vi "FuzzyEx User-defined Membership Functions.vi"() -> ()   [LabVIEW 2023]
doc: "This VI demonstrates how to create your own user-defined membership function and use the API to evaluate a system by using the new membership function."
uses:
  <vilib>/addons/Fuzzy Logic/TypeDefs/FL Modifier.ctl
  <vilib>/addons/Fuzzy Logic/TypeDefs/FL Antecedent Connective.ctl
  <vilib>/addons/Fuzzy Logic/TypeDefs/FL Consequent Implication.ctl
  <vilib>/addons/Fuzzy Logic/Membership/FL Create Membership Function (User-Defined).vi
  <vilib>/addons/Fuzzy Logic/FL Fuzzy Controller (SISO).vi
  <vilib>/addons/Fuzzy Logic/NI_Fuzzy_Logic_API.lvlib
panel:
  in  "Overview":string="Overview: This VI demonstrates how to create your own user-defined membership function and use the API to evaluate a system by using the new membership function.\nInstructions:\n1. Run the VI.\n2. Change shape by moving the Basic Membership Shape cursors or directly changing values in the cursor table. Keep in mind the X and Y arrays must contain elements in ascending order for convenient interpolation results. \n3. Move the slider below the Membership Function graph to evaluate the membership grade.\n4. Change the left base, left top, right top and right base values to modify the range of the function.\n5. Click Stop to stop the VI."
  out "Error":bool
  in  "Basic Membership Shape":cluster{cluster{"Xi":dbl, "Yi":dbl}[]}[](graph)=[{[{"Xi"=-8.0, "Yi"=0.0}, {"Xi"=-7.919597989949748, "Yi"=0.04719031897891056}, {"Xi"=-7.839195979899498, "Yi"=0.0936509941538288}, {"Xi"=-7.758793969849246, "Yi"=0.13877501021805186}, {"Xi"=-7.678391959798995, "Yi"=0.18195535186487483}, {"Xi"=-7.597989949748744, "Yi"=0.22258500378759477}, {"Xi"=-7.517587939698492, "Yi"=0.26039081912974815}, {"Xi"=-7.437185929648241, "Yi"=0.29776297115463546}, {"Xi"=-7.35678391959799, "Yi"=0.3351151121007157}, {"Xi"=-7.276381909547739, "Yi"=0.37222372887356214}, {"Xi"=-7.1959798994974875, "Yi"=0.4088653083787497}, {"Xi"=-7.115577889447236, "Yi"=0.44481633752185185}, {"Xi"=-7.035175879396985, "Yi"=0.4798533032084424}, {"Xi"=-6.954773869346734, "Yi"=0.513752692344096}, {"Xi"=-6.874371859296482, "Yi"=0.5462909918343865}, {"Xi"=-6.793969849246231, "Yi"=0.5772446885848874}, {"Xi"=-6.71356783919598, "Yi"=0.6063902695011735}, {"Xi"=-6.633165829145729, "Yi"=0.6335042214888181}, {"Xi"=-6.552763819095477, "Yi"=0.6583630314533961}, {"Xi"=-6.472361809045226, "Yi"=0.6807431863004809}, {"Xi"=-6.391959798994975, "Yi"=0.7004211729356467}, {"Xi"=-6.311557788944723, "Yi"=0.7172252080175027}, {"Xi"=-6.231155778894473, "Yi"=0.7329213118498933}, {"Xi"=-6.150753768844221, "Yi"=0.7484474478322185}, {"Xi"=-6.0703517587939695, "Yi"=0.7637753085739313}, {"Xi"=-5.989949748743719, "Yi"=0.7788765866844846}, {"Xi"=-5.909547738693467, "Yi"=0.7937229747733321}, {"Xi"=-5.8291457286432165, "Yi"=0.8082861654499267}, {"Xi"=-5.748743718592965, "Yi"=0.8225378513237219}, {"Xi"=-5.668341708542713, "Yi"=0.8364497250041708}, {"Xi"=-5.5879396984924625, "Yi"=0.8499934791007266}, {"Xi"=-5.507537688442211, "Yi"=0.8631408062228427}, {"Xi"=-5.42713567839196, "Yi"=0.875863398979972}, {"Xi"=-5.346733668341709, "Yi"=0.8881329499815682}, {"Xi"=-5.266331658291457, "Yi"=0.8999211518370842}, {"Xi"=-5.185929648241206, "Yi"=0.9111996971559733}, {"Xi"=-5.105527638190955, "Yi"=0.9219402785476887}, {"Xi"=-5.025125628140704, "Yi"=0.9321145886216837}, {"Xi"=-4.944723618090452, "Yi"=0.9416943199874116}, {"Xi"=-4.864321608040201, "Yi"=0.9506511652543255}, {"Xi"=-4.78391959798995, "Yi"=0.9589568170318786}, {"Xi"=-4.703517587939698, "Yi"=0.9665829679295244}, {"Xi"=-4.623115577889447, "Yi"=0.9735013105567158}, {"Xi"=-4.542713567839196, "Yi"=0.9796835375229063}, {"Xi"=-4.4623115577889445, "Yi"=0.985101341437549}, {"Xi"=-4.381909547738694, "Yi"=0.989726414910097}, {"Xi"=-4.301507537688442, "Yi"=0.993530450550004}, {"Xi"=-4.221105527638191, "Yi"=0.9964851409667227}, {"Xi"=-4.14070351758794, "Yi"=0.9985621787697065}, {"Xi"=-4.060301507537688, "Yi"=0.9997332565684088}, {"Xi"=-3.979899497487437, "Yi"=1.0}, {"Xi"=-3.899497487437186, "Yi"=1.0}, {"Xi"=-3.819095477386935, "Yi"=1.0}, {"Xi"=-3.7386934673366836, "Yi"=1.0}, {"Xi"=-3.658291457286432, "Yi"=1.0}, {"Xi"=-3.577889447236181, "Yi"=1.0}, {"Xi"=-3.4974874371859297, "Yi"=1.0}, {"Xi"=-3.4170854271356785, "Yi"=1.0}, {"Xi"=-3.336683417085427, "Yi"=1.0}, {"Xi"=-3.2562814070351758, "Yi"=1.0}, {"Xi"=-3.1758793969849246, "Yi"=1.0}, {"Xi"=-3.0954773869346734, "Yi"=1.0}, {"Xi"=-3.0150753768844223, "Yi"=1.0}, {"Xi"=-2.9346733668341707, "Yi"=1.0}, {"Xi"=-2.8542713567839195, "Yi"=1.0}, {"Xi"=-2.7738693467336684, "Yi"=1.0}, {"Xi"=-2.693467336683417, "Yi"=1.0}, {"Xi"=-2.613065326633166, "Yi"=1.0}, {"Xi"=-2.5326633165829144, "Yi"=1.0}, {"Xi"=-2.4522613065326633, "Yi"=1.0}, {"Xi"=-2.371859296482412, "Yi"=1.0}, {"Xi"=-2.291457286432161, "Yi"=1.0}, {"Xi"=-2.2110552763819094, "Yi"=1.0}, {"Xi"=-2.130653266331658, "Yi"=1.0}, {"Xi"=-2.050251256281407, "Yi"=1.0}, {"Xi"=-1.9698492462311559, "Yi"=1.0}, {"Xi"=-1.8894472361809045, "Yi"=1.0}, {"Xi"=-1.8090452261306533, "Yi"=1.0}, {"Xi"=-1.728643216080402, "Yi"=1.0}, {"Xi"=-1.6482412060301508, "Yi"=1.0}, {"Xi"=-1.5678391959798994, "Yi"=1.0}, {"Xi"=-1.4874371859296482, "Yi"=1.0}, {"Xi"=-1.407035175879397, "Yi"=1.0}, {"Xi"=-1.3266331658291457, "Yi"=1.0}, {"Xi"=-1.2462311557788945, "Yi"=1.0}, {"Xi"=-1.1658291457286432, "Yi"=1.0}, {"Xi"=-1.085427135678392, "Yi"=1.0}, {"Xi"=-1.0050251256281406, "Yi"=1.0}, {"Xi"=-0.9246231155778895, "Yi"=1.0}, {"Xi"=-0.8442211055276382, "Yi"=1.0}, {"Xi"=-0.7638190954773869, "Yi"=1.0}, {"Xi"=-0.6834170854271356, "Yi"=1.0}, {"Xi"=-0.6030150753768844, "Yi"=1.0}, {"Xi"=-0.5226130653266332, "Yi"=1.0}, {"Xi"=-0.44221105527638194, "Yi"=1.0}, {"Xi"=-0.36180904522613067, "Yi"=1.0}, {"Xi"=-0.2814070351758794, "Yi"=1.0}, {"Xi"=-0.20100502512562815, "Yi"=1.0}, {"Xi"=-0.12060301507537688, "Yi"=1.0}, {"Xi"=-0.04020100502512563, "Yi"=1.0}, {"Xi"=0.04020100502512563, "Yi"=1.0}, {"Xi"=0.12060301507537688, "Yi"=1.0}, {"Xi"=0.20100502512562815, "Yi"=1.0}, {"Xi"=0.2814070351758794, "Yi"=1.0}, {"Xi"=0.36180904522613067, "Yi"=1.0}, {"Xi"=0.44221105527638194, "Yi"=1.0}, {"Xi"=0.5226130653266332, "Yi"=1.0}, {"Xi"=0.6030150753768844, "Yi"=1.0}, {"Xi"=0.6834170854271356, "Yi"=1.0}, {"Xi"=0.7638190954773869, "Yi"=1.0}, {"Xi"=0.8442211055276382, "Yi"=1.0}, {"Xi"=0.9246231155778895, "Yi"=1.0}, {"Xi"=1.0050251256281406, "Yi"=0.999999390841234}, {"Xi"=1.085427135678392, "Yi"=0.9998249469013698}, {"Xi"=1.1658291457286432, "Yi"=0.9993441155957051}, {"Xi"=1.2462311557788945, "Yi"=0.9985621787697065}, {"Xi"=1.3266331658291457, "Yi"=0.9974844182688406}, {"Xi"=1.407035175879397, "Yi"=0.9961161159385735}, {"Xi"=1.4874371859296482, "Yi"=0.994462553624372}, {"Xi"=1.5678391959798994, "Yi"=0.9925290131717022}, {"Xi"=1.6482412060301508, "Yi"=0.9903207764260309}, {"Xi"=1.728643216080402, "Yi"=0.9878431252328242}, {"Xi"=1.8090452261306533, "Yi"=0.985101341437549}, {"Xi"=1.8894472361809045, "Yi"=0.9821007068856714}, {"Xi"=1.9698492462311559, "Yi"=0.9788465034226579}, {"Xi"=2.050251256281407, "Yi"=0.975344012893975}, {"Xi"=2.130653266331658, "Yi"=0.9715985171450893}, {"Xi"=2.2110552763819094, "Yi"=0.967615298021467}, {"Xi"=2.291457286432161, "Yi"=0.9633996373685746}, {"Xi"=2.371859296482412, "Yi"=0.9589568170318786}, {"Xi"=2.4522613065326633, "Yi"=0.9542921188568456}, {"Xi"=2.5326633165829144, "Yi"=0.9494108246889419}, {"Xi"=2.613065326633166, "Yi"=0.9443182163736339}, {"Xi"=2.693467336683417, "Yi"=0.9390195757563881}, {"Xi"=2.7738693467336684, "Yi"=0.9335201846826711}, {"Xi"=2.8542713567839195, "Yi"=0.927825324997949}, {"Xi"=2.9346733668341707, "Yi"=0.9219402785476887}, {"Xi"=3.0150753768844223, "Yi"=0.9158703271773563}, {"Xi"=3.0954773869346734, "Yi"=0.9096207527324184}, {"Xi"=3.1758793969849246, "Yi"=0.9031968370583415}, {"Xi"=3.2562814070351758, "Yi"=0.896603862000592}, {"Xi"=3.336683417085427, "Yi"=0.8898471094046363}, {"Xi"=3.4170854271356785, "Yi"=0.8829318611159407}, {"Xi"=3.4974874371859297, "Yi"=0.8758633989799721}, {"Xi"=3.577889447236181, "Yi"=0.8686470048421966}, {"Xi"=3.658291457286432, "Yi"=0.8612879605480808}, {"Xi"=3.7386934673366836, "Yi"=0.8537915479430909}, {"Xi"=3.819095477386935, "Yi"=0.8461630488726938}, {"Xi"=3.899497487437186, "Yi"=0.8384077451823555}, {"Xi"=3.979899497487437, "Yi"=0.8305309187175428}, {"Xi"=4.060301507537688, "Yi"=0.8225378513237219}, {"Xi"=4.14070351758794, "Yi"=0.8144338248463594}, {"Xi"=4.221105527638191, "Yi"=0.8062241211309217}, {"Xi"=4.301507537688442, "Yi"=0.7979140220228752}, {"Xi"=4.381909547738694, "Yi"=0.7895088093676864}, {"Xi"=4.4623115577889445, "Yi"=0.781013765010822}, {"Xi"=4.542713567839196, "Yi"=0.772434170797748}, {"Xi"=4.623115577889447, "Yi"=0.7637753085739312}, {"Xi"=4.703517587939698, "Yi"=0.7550424601848378}, {"Xi"=4.78391959798995, "Yi"=0.7462409074759343}, {"Xi"=4.864321608040201, "Yi"=0.7373759322926875}, {"Xi"=4.944723618090452, "Yi"=0.7284528164805634}, {"Xi"=5.025125628140704, "Yi"=0.7194768418850286}, {"Xi"=5.105527638190955, "Yi"=0.7103665016452464}, {"Xi"=5.185929648241206, "Yi"=0.7004211729356467}, {"Xi"=5.266331658291457, "Yi"=0.6895205197178526}, {"Xi"=5.346733668341709, "Yi"=0.6777062470590457}, {"Xi"=5.42713567839196, "Yi"=0.6650200600264075}, {"Xi"=5.507537688442211, "Yi"=0.6515036636871199}, {"Xi"=5.5879396984924625, "Yi"=0.6371987631083638}, {"Xi"=5.668341708542713, "Yi"=0.6221470633573212}, {"Xi"=5.748743718592965, "Yi"=0.6063902695011734}, {"Xi"=5.8291457286432165, "Yi"=0.5899700866071019}, {"Xi"=5.909547738693467, "Yi"=0.5729282197422885}, {"Xi"=5.989949748743719, "Yi"=0.5553063739739142}, {"Xi"=6.0703517587939695, "Yi"=0.5371462543691613}, {"Xi"=6.150753768844221, "Yi"=0.5184895659952105}, {"Xi"=6.231155778894473, "Yi"=0.49937801391924364}, {"Xi"=6.311557788944723, "Yi"=0.47985330320844255}, {"Xi"=6.391959798994975, "Yi"=0.45995713892998824}, {"Xi"=6.472361809045226, "Yi"=0.4397312261510627}, {"Xi"=6.552763819095477, "Yi"=0.419217269938847}, {"Xi"=6.633165829145729, "Yi"=0.3984569753605229}, {"Xi"=6.71356783919598, "Yi"=0.37749204748327214}, {"Xi"=6.793969849246231, "Yi"=0.3563641913742757}, {"Xi"=6.874371859296482, "Yi"=0.33511511210071576}, {"Xi"=6.954773869346734, "Yi"=0.31378651472977315}, {"Xi"=7.035175879396985, "Yi"=0.2924201043286298}, {"Xi"=7.115577889447236, "Yi"=0.2710575859644674}, {"Xi"=7.1959798994974875, "Yi"=0.24974066470446693}, {"Xi"=7.276381909547739, "Yi"=0.22814562572871505}, {"Xi"=7.35678391959799, "Yi"=0.2055235591010643}, {"Xi"=7.437185929648241, "Yi"=0.18195535186487494}, {"Xi"=7.517587939698492, "Yi"=0.1575542663514276}, {"Xi"=7.597989949748744, "Yi"=0.13243356489200173}, {"Xi"=7.678391959798995, "Yi"=0.1067065098178776}, {"Xi"=7.758793969849246, "Yi"=0.08048636346033558}, {"Xi"=7.839195979899498, "Yi"=0.053886388150655086}, {"Xi"=7.919597989949748, "Yi"=0.027019846220116755}, {"Xi"=8.0, "Yi"=0.0}]}]
  in  "Stop":bool
  out "Membership grade":dbl(slide)=0.6596021514020028 scale=0.0..1.0
  in  "input value":dbl(slide)=4.535315985130112 scale=-10.0..10.0
  out "Membership function":cluster{cluster{"Xi":dbl, "Yi":dbl}[]}[](graph)=[{[{"Xi"=-8.0, "Yi"=0.0}, {"Xi"=-7.919597989949748, "Yi"=0.04525637619716676}, {"Xi"=-7.839195979899498, "Yi"=0.089101739755963}, {"Xi"=-7.758793969849246, "Yi"=0.13147220499791226}, {"Xi"=-7.678391959798995, "Yi"=0.17230388624453624}, {"Xi"=-7.597989949748744, "Yi"=0.21153289781735835}, {"Xi"=-7.517587939698492, "Yi"=0.24909535403790078}, {"Xi"=-7.437185929648241, "Yi"=0.2849273692276857}, {"Xi"=-7.35678391959799, "Yi"=0.3189650577082365}, {"Xi"=-7.276381909547739, "Yi"=0.351144533801075}, {"Xi"=-7.1959798994974875, "Yi"=0.38140191182772454}, {"Xi"=-7.115577889447236, "Yi"=0.40967330610970726}, {"Xi"=-7.035175879396985, "Yi"=0.4358948309685456}, {"Xi"=-6.954773869346734, "Yi"=0.46000260072576254}, {"Xi"=-6.874371859296482, "Yi"=0.4819165744611297}, {"Xi"=-6.793969849246231, "Yi"=0.5016954632128382}, {"Xi"=-6.71356783919598, "Yi"=0.5197150776642824}, {"Xi"=-6.633165829145729, "Yi"=0.5363726915150068}, {"Xi"=-6.552763819095477, "Yi"=0.5520655784645572}, {"Xi"=-6.472361809045226, "Yi"=0.5671910122124783}, {"Xi"=-6.391959798994975, "Yi"=0.5821462664583151}, {"Xi"=-6.311557788944723, "Yi"=0.5973286149016133}, {"Xi"=-6.231155778894473, "Yi"=0.6131353312419173}, {"Xi"=-6.150753768844221, "Yi"=0.629955017725542}, {"Xi"=-6.0703517587939695, "Yi"=0.6479014267980455}, {"Xi"=-5.989949748743719, "Yi"=0.6668179425698928}, {"Xi"=-5.909547738693467, "Yi"=0.686538545391848}, {"Xi"=-5.8291457286432165, "Yi"=0.7068972156146747}, {"Xi"=-5.748743718592965, "Yi"=0.7277279335891373}, {"Xi"=-5.668341708542713, "Yi"=0.7488646796659998}, {"Xi"=-5.5879396984924625, "Yi"=0.7701414341960257}, {"Xi"=-5.507537688442211, "Yi"=0.7913921775299795}, {"Xi"=-5.42713567839196, "Yi"=0.8124508900186247}, {"Xi"=-5.346733668341709, "Yi"=0.8331515520127257}, {"Xi"=-5.266331658291457, "Yi"=0.8533281438630463}, {"Xi"=-5.185929648241206, "Yi"=0.8728146459203504}, {"Xi"=-5.105527638190955, "Yi"=0.8914450385354021}, {"Xi"=-5.025125628140704, "Yi"=0.9090533020589653}, {"Xi"=-4.944723618090452, "Yi"=0.9254734168418042}, {"Xi"=-4.864321608040201, "Yi"=0.9405393632346825}, {"Xi"=-4.78391959798995, "Yi"=0.9540851215883641}, {"Xi"=-4.703517587939698, "Yi"=0.9659446722536132}, {"Xi"=-4.623115577889447, "Yi"=0.9759519955811939}, {"Xi"=-4.542713567839196, "Yi"=0.9839410719218699}, {"Xi"=-4.4623115577889445, "Yi"=0.9897458816264053}, {"Xi"=-4.381909547738694, "Yi"=0.9932004074607601}, {"Xi"=-4.301507537688442, "Yi"=0.9953659353767574}, {"Xi"=-4.221105527638191, "Yi"=0.9972948938536792}, {"Xi"=-4.14070351758794, "Yi"=0.9988182838797}, {"Xi"=-4.060301507537688, "Yi"=0.9997671064429944}, {"Xi"=-3.979899497487437, "Yi"=1.0}, {"Xi"=-3.899497487437186, "Yi"=1.0}, {"Xi"=-3.819095477386935, "Yi"=1.0}, {"Xi"=-3.7386934673366836, "Yi"=1.0}, {"Xi"=-3.658291457286432, "Yi"=1.0}, {"Xi"=-3.577889447236181, "Yi"=1.0}, {"Xi"=-3.4974874371859297, "Yi"=1.0}, {"Xi"=-3.4170854271356785, "Yi"=1.0}, {"Xi"=-3.336683417085427, "Yi"=1.0}, {"Xi"=-3.2562814070351758, "Yi"=1.0}, {"Xi"=-3.1758793969849246, "Yi"=1.0}, {"Xi"=-3.0954773869346734, "Yi"=1.0}, {"Xi"=-3.0150753768844223, "Yi"=1.0}, {"Xi"=-2.9346733668341707, "Yi"=1.0}, {"Xi"=-2.8542713567839195, "Yi"=1.0}, {"Xi"=-2.7738693467336684, "Yi"=1.0}, {"Xi"=-2.693467336683417, "Yi"=1.0}, {"Xi"=-2.613065326633166, "Yi"=1.0}, {"Xi"=-2.5326633165829144, "Yi"=1.0}, {"Xi"=-2.4522613065326633, "Yi"=1.0}, {"Xi"=-2.371859296482412, "Yi"=1.0}, {"Xi"=-2.291457286432161, "Yi"=1.0}, {"Xi"=-2.2110552763819094, "Yi"=1.0}, {"Xi"=-2.130653266331658, "Yi"=1.0}, {"Xi"=-2.050251256281407, "Yi"=1.0}, {"Xi"=-1.9698492462311559, "Yi"=1.0}, {"Xi"=-1.8894472361809045, "Yi"=1.0}, {"Xi"=-1.8090452261306533, "Yi"=1.0}, {"Xi"=-1.728643216080402, "Yi"=1.0}, {"Xi"=-1.6482412060301508, "Yi"=1.0}, {"Xi"=-1.5678391959798994, "Yi"=1.0}, {"Xi"=-1.4874371859296482, "Yi"=1.0}, {"Xi"=-1.407035175879397, "Yi"=1.0}, {"Xi"=-1.3266331658291457, "Yi"=1.0}, {"Xi"=-1.2462311557788945, "Yi"=1.0}, {"Xi"=-1.1658291457286432, "Yi"=1.0}, {"Xi"=-1.085427135678392, "Yi"=1.0}, {"Xi"=-1.0050251256281406, "Yi"=1.0}, {"Xi"=-0.9246231155778895, "Yi"=1.0}, {"Xi"=-0.8442211055276382, "Yi"=1.0}, {"Xi"=-0.7638190954773869, "Yi"=1.0}, {"Xi"=-0.6834170854271356, "Yi"=1.0}, {"Xi"=-0.6030150753768844, "Yi"=1.0}, {"Xi"=-0.5226130653266332, "Yi"=1.0}, {"Xi"=-0.44221105527638194, "Yi"=1.0}, {"Xi"=-0.36180904522613067, "Yi"=1.0}, {"Xi"=-0.2814070351758794, "Yi"=1.0}, {"Xi"=-0.20100502512562815, "Yi"=1.0}, {"Xi"=-0.12060301507537688, "Yi"=1.0}, {"Xi"=-0.04020100502512563, "Yi"=1.0}, {"Xi"=0.04020100502512563, "Yi"=1.0}, {"Xi"=0.12060301507537688, "Yi"=1.0}, {"Xi"=0.20100502512562815, "Yi"=1.0}, {"Xi"=0.2814070351758794, "Yi"=1.0}, {"Xi"=0.36180904522613067, "Yi"=1.0}, {"Xi"=0.44221105527638194, "Yi"=1.0}, {"Xi"=0.5226130653266332, "Yi"=1.0}, {"Xi"=0.6030150753768844, "Yi"=1.0}, {"Xi"=0.6834170854271356, "Yi"=1.0}, {"Xi"=0.7638190954773869, "Yi"=1.0}, {"Xi"=0.8442211055276382, "Yi"=1.0}, {"Xi"=0.9246231155778895, "Yi"=1.0}, {"Xi"=1.0050251256281406, "Yi"=0.9999994462347956}, {"Xi"=1.085427135678392, "Yi"=0.9998458948873343}, {"Xi"=1.1658291457286432, "Yi"=0.9994416629878643}, {"Xi"=1.2462311557788945, "Yi"=0.9988182838797}, {"Xi"=1.3266331658291457, "Yi"=0.9980072909061556}, {"Xi"=1.407035175879397, "Yi"=0.9970402174105455}, {"Xi"=1.4874371859296482, "Yi"=0.9959485967361842}, {"Xi"=1.5678391959798994, "Yi"=0.9947639622263859}, {"Xi"=1.6482412060301508, "Yi"=0.9935178472244648}, {"Xi"=1.728643216080402, "Yi"=0.9920183336567963}, {"Xi"=1.8090452261306533, "Yi"=0.9897458816264053}, {"Xi"=1.8894472361809045, "Yi"=0.9867059891762994}, {"Xi"=1.9698492462311559, "Yi"=0.9829296337337414}, {"Xi"=2.050251256281407, "Yi"=0.978447792725994}, {"Xi"=2.130653266331658, "Yi"=0.9732914435803198}, {"Xi"=2.2110552763819094, "Yi"=0.9674915637239817}, {"Xi"=2.291457286432161, "Yi"=0.9610791305842422}, {"Xi"=2.371859296482412, "Yi"=0.9540851215883641}, {"Xi"=2.4522613065326633, "Yi"=0.94654051416361}, {"Xi"=2.5326633165829144, "Yi"=0.9384762857372427}, {"Xi"=2.613065326633166, "Yi"=0.9299234137365249}, {"Xi"=2.693467336683417, "Yi"=0.9209128755887191}, {"Xi"=2.7738693467336684, "Yi"=0.9114756487210883}, {"Xi"=2.8542713567839195, "Yi"=0.9016427105608951}, {"Xi"=2.9346733668341707, "Yi"=0.8914450385354021}, {"Xi"=3.0150753768844223, "Yi"=0.880913610071872}, {"Xi"=3.0954773869346734, "Yi"=0.8700794025975676}, {"Xi"=3.1758793969849246, "Yi"=0.8589733935397517}, {"Xi"=3.2562814070351758, "Yi"=0.8476265603256866}, {"Xi"=3.336683417085427, "Yi"=0.8360698803826353}, {"Xi"=3.4170854271356785, "Yi"=0.8243343311378604}, {"Xi"=3.4974874371859297, "Yi"=0.8124508900186248}, {"Xi"=3.577889447236181, "Yi"=0.8004505344521909}, {"Xi"=3.658291457286432, "Yi"=0.7883642418658215}, {"Xi"=3.7386934673366836, "Yi"=0.7762229896867794}, {"Xi"=3.819095477386935, "Yi"=0.7640577553423273}, {"Xi"=3.899497487437186, "Yi"=0.7518995162597277}, {"Xi"=3.979899497487437, "Yi"=0.7397792498662435}, {"Xi"=4.060301507537688, "Yi"=0.7277279335891373}, {"Xi"=4.14070351758794, "Yi"=0.7157765448556719}, {"Xi"=4.221105527638191, "Yi"=0.7039560610931099}, {"Xi"=4.301507537688442, "Yi"=0.6922974597287139}, {"Xi"=4.381909547738694, "Yi"=0.6808317181897467}, {"Xi"=4.4623115577889445, "Yi"=0.6695898139034713}, {"Xi"=4.542713567839196, "Yi"=0.6586027242971499}, {"Xi"=4.623115577889447, "Yi"=0.6479014267980455}, {"Xi"=4.703517587939698, "Yi"=0.6375168988334206}, {"Xi"=4.78391959798995, "Yi"=0.627480117830538}, {"Xi"=4.864321608040201, "Yi"=0.6178218108816823}, {"Xi"=4.944723618090452, "Yi"=0.6085322509161566}, {"Xi"=5.025125628140704, "Yi"=0.5995392247711216}, {"Xi"=5.105527638190955, "Yi"=0.5907686055755252}, {"Xi"=5.185929648241206, "Yi"=0.5821462664583151}, {"Xi"=5.266331658291457, "Yi"=0.5735980805484393}, {"Xi"=5.346733668341709, "Yi"=0.5650499209748455}, {"Xi"=5.42713567839196, "Yi"=0.5564276608664815}, {"Xi"=5.507537688442211, "Yi"=0.5476571733522956}, {"Xi"=5.5879396984924625, "Yi"=0.538664331561235}, {"Xi"=5.668341708542713, "Yi"=0.5293750086222481}, {"Xi"=5.748743718592965, "Yi"=0.5197150776642823}, {"Xi"=5.8291457286432165, "Yi"=0.5096104118162856}, {"Xi"=5.909547738693467, "Yi"=0.49898688420720616}, {"Xi"=5.989949748743719, "Yi"=0.4877703679659914}, {"Xi"=6.0703517587939695, "Yi"=0.47588673622158945}, {"Xi"=6.150753768844221, "Yi"=0.46327029128462166}, {"Xi"=6.231155778894473, "Yi"=0.44993362418023397}, {"Xi"=6.311557788944723, "Yi"=0.4358948309685457}, {"Xi"=6.391959798994975, "Yi"=0.42116583200938895}, {"Xi"=6.472361809045226, "Yi"=0.4057585476625966}, {"Xi"=6.552763819095477, "Yi"=0.3896848982880009}, {"Xi"=6.633165829145729, "Yi"=0.3729568042454345}, {"Xi"=6.71356783919598, "Yi"=0.35558618589473007}, {"Xi"=6.793969849246231, "Yi"=0.33758496359571977}, {"Xi"=6.874371859296482, "Yi"=0.3189650577082365}, {"Xi"=6.954773869346734, "Yi"=0.29973838859211244}, {"Xi"=7.035175879396985, "Yi"=0.27991687660718023}, {"Xi"=7.115577889447236, "Yi"=0.25951244211327273}, {"Xi"=7.1959798994974875, "Yi"=0.23853700547022186}, {"Xi"=7.276381909547739, "Yi"=0.2170024870378605}, {"Xi"=7.35678391959799, "Yi"=0.1949208071760213}, {"Xi"=7.437185929648241, "Yi"=0.17230388624453635}, {"Xi"=7.517587939698492, "Yi"=0.14916364460323867}, {"Xi"=7.597989949748744, "Yi"=0.12551200261196027}, {"Xi"=7.678391959798995, "Yi"=0.10136088063053392}, {"Xi"=7.758793969849246, "Yi"=0.07672219901879242}, {"Xi"=7.839195979899498, "Yi"=0.051607878136567725}, {"Xi"=7.919597989949748, "Yi"=0.026029838343692942}, {"Xi"=8.0, "Yi"=0.0}]}]
  in  "right base":dbl=8.0
  in  "right top":dbl=1.0
  in  "left top":dbl=-4.0
  in  "left base":dbl=-8.0
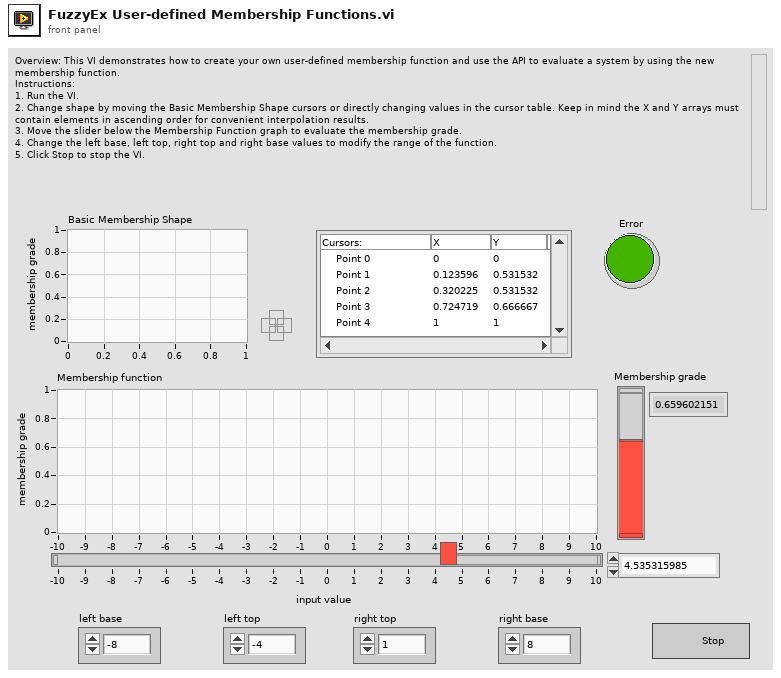
[diagram p1: front panel]
types:
  T1 = typedef "NI_Fuzzy_Logic_API.lvlib/FL Consequent Implication.ctl" = u16
  T2 = typedef "NI_Fuzzy_Logic_API.lvlib/FL Antecedent Connective.ctl" = u16
  T3 = typedef "NI_Fuzzy_Logic_API.lvlib/FL Modifier.ctl" = u16
  T4 = typedef "NI_Fuzzy_Logic_API.lvlib/FL Antecedent.ctl" = cluster{"Var Index":i32, "MF Index":i32, "Cond":T3}
  T5 = typedef "NI_Fuzzy_Logic_API.lvlib/FL Consequent.ctl" = cluster{"Var Index":i32, "MF Index":i32, "Cond":T3}
  T6 = typedef "LVCursorListTypeDef.ctl" = cluster{"Name":string, "Color":u32, "Style":u8, "Point Style":u8, "Name Visible":bool, "Allow Drag":bool, "Cursor Mode":u32, "Plot":i32, "Index":i32, "Position":cluster{"X":dbl, "Y":dbl}, "X Scale":u32, "Y Scale":u32, "Watch Plots":i32[], "Watch All Plots":bool, "Plot Area":i32, "Label Offset":cluster{"X":dbl, "Y":dbl}}[]
  T7 = typedef "NI_Fuzzy_Logic_API.lvlib/FL Rule.ctl" = cluster{"antecedents":T4[], "antecedent connective":T2, "consequents":T5[], "consequent implication":T1, "degree of support":dbl}
  T8 = typedef "NI_Fuzzy_Logic_API.lvlib/FL Membership Function.ctl" = cluster{"name":string, "shape":T9, "points":dbl[], "color":u32, "user-defined shape index":i32}
  T9 = typedef "NI_Fuzzy_Logic_API.lvlib/FL Membership Function Shape.ctl" = u16
  T10 = typedef "NI_Fuzzy_Logic_API.lvlib/FL Variable.ctl" = cluster{"name":string, "range":dbl[], "MFs":T8[]}
  T11 = typedef "NI_Fuzzy_Logic_API.lvlib/FL System.ctl" = cluster{"input variables":T10[], "output variables":T10[], "rules":T7[], "defuzzification method":T12, "description":string, "user MF interpolating polynomials":T13[]}
  T12 = typedef "NI_Fuzzy_Logic_API.lvlib/FL Defuzzification.ctl" = u16
  T13 = typedef "NI_Fuzzy_Logic_API.lvlib/FL Interpolating polynomials.ctl" = cluster{"X":dbl[], "Y":dbl[], "Y(x) coeff":dbl[][], "X(y) coeff":dbl[][], "Area(y) coeff":dbl[][], "coa_x(y) coeff":dbl[][]}
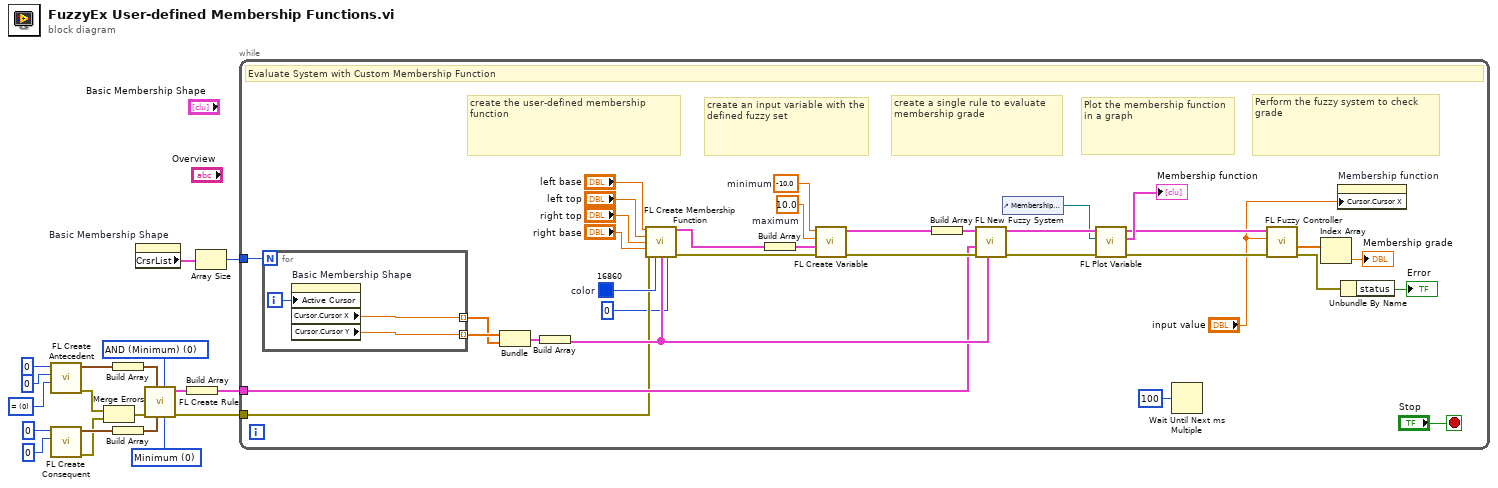
[diagram p0: block diagram]
diagram:
  w9 = T1 0 items=["Minimum", "Product"] ("consequent implication")
  w10 = T2 0 items=["AND (Minimum)", "AND (Product)", "OR (Maximum)", "OR (Probabilistic)"] ("antecedent connective")
  w19 = T3 0 items=["=", "!="] ("condition")
  n1 = call <vilib>:"FL Create Antecedent.vi"("condition"=w19, "membership function index"=0, "variable index"=0) -> ("error out"=w4:errorcluster, "antecedent"=w15:T4)  [unwired: 7 in]
  n2 = call <vilib>:"FL Create Consequent.vi"("membership function index"=0, "variable index"=0) -> ("error out"=w3:errorcluster, "consequent"=w14:T5)  [unwired: 8 in]
  n3 = Merge Errors(w4, w3) -> (w5:errorcluster)
  n4 = Build Array(w15) -> (w13:T4[])
  n5 = Build Array(w14) -> (w12:T5[])
  n6 = property on="Basic Membership Shape" class="XYGraph (strict)"() -> ("CrsrList"=w8:T6)  [unwired: 2 in, 2 out]
  n7 = call <vilib>:"FL Create Rule.vi"("consequent implication"=w9, "antecedent connective"=w10, "consequents"=w12, "antecedents"=w13, "error in (no error)"=w5) -> ("error out"=w2:errorcluster, "rule"=w11:T7)  [unwired: 5 in]
  n8 = Build Array(w11) -> (w6:T7[])
  n9 = Array Size(array=w8) -> (size(s)=w7:i32)
  n10 = while {
    tunnel: w7 -> [w27]
    tunnel: w6 -> [w22]
    tunnel: w2 -> [w21]
    stop <- "Stop" stop-if-true
    w41 = 10.0  # maximum
    w42 = -10.0  # minimum
    w43 = u32 16860  # color
    # "Perform the fuzzy system to check grade"
    # "Plot the membership function in a graph"
    # "create a single rule to evaluate membership grade"
    # "create an input variable with the defined fuzzy set"
    # "create the user-defined membership function"
    # "Evaluate System with Custom Membership Function"
    n11 = for {
      N: w27 -> [_]
      tunnel: [w56] -> w25 mode=indexing
      tunnel: [w55] -> w26 mode=indexing
      i -> [w54]
      n12 = property on="Basic Membership Shape" class="XYGraph (strict)"("Active Cursor"=w54) -> ("Cursor.Cursor X"=w56:dbl, "Cursor.Cursor Y"=w55:dbl)  [unwired: 2 in, 2 out]
    }
    n13 = Bundle(w26, w25) -> (w30:cluster{dbl[], dbl[]})  [unwired: 1 in]
    n14 = Build Array(w30) -> (w29:cluster{dbl[], dbl[]}[])
    n15 = call-poly <vilib>:"FL Create Membership Function.vi"("left base"="left base", "left top"="left top", "right top"="right top", "right base"="right base", "error in (no error)"=w21, "color"=w43, "user-defined membership function shapes"=w29, "user-defined shape index"=0) -> ("membership function"=w53:T8, "error out"=w48:errorcluster)  [unwired: 6 in]
    n16 = Build Array(w53) -> (w52:T8[])
    n17 = call <vilib>:"FL Create Variable.vi"("error in (no error)"=w48, "membership functions"=w52, "maximum"=w41, "minimum"=w42) -> ("error out"=w49:errorcluster, "variable"=w51:T10)  [unwired: 6 in]
    n18 = Build Array(w51) -> (w50:T10[])
    n19 = call <vilib>:"FL New Fuzzy System.vi"("user-defined membership function shapes"=w29, "error in (no error)"=w49, "rules"=w22, "input variables"=w50) -> ("error out"=w39:errorcluster, "fuzzy system out"=w38:T11)  [unwired: 6 in]
    n20 = control-ref of="Membership function"() -> (w28:refnum<vi>)
    n21 = call <vilib>:"FL Plot Variable.vi"("error in (no error)"=w39, "graph refnum"=w28, "fuzzy system in"=w38) -> ("error out"=w34:errorcluster, "membership functions plot"=→"Membership function":cluster{cluster{"Xi":dbl, "Yi":dbl}[]}[], "fuzzy system out"=w35:T11)  [unwired: 6 in]
    n22 = Wait Until Next ms Multiple(millisecond multiple=u32 100) -> ()  [unwired: 1 out]
    n23 = call-poly <vilib>:"FL Fuzzy Controller.vi"("error in (no error)"=w34, "input value"="input value", "fuzzy system in"=w35) -> ("error out"=w24:errorcluster, "rule weights"=w37:dbl[])  [unwired: 4 in, 3 out]
    n24 = Index Array(array=w37) -> (element=→"Membership grade":dbl)  [unwired: 1 in]
    n25 = property on="Membership function" class="XYGraph (strict)"("Cursor.Cursor X"="input value") -> ()  [unwired: 2 in, 2 out]
    n26 = Unbundle By Name(w24) -> ("status"=→"Error":bool)
  }
